vi "FMS Data Array.vi"() -> (0 "FMS Data Array":string[](array[string]), 2 "Scale":string, 3 "Switch":string)   [LabVIEW 2017]
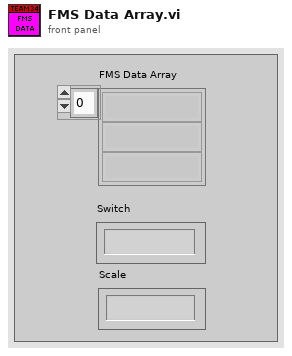
[diagram p1: front panel]
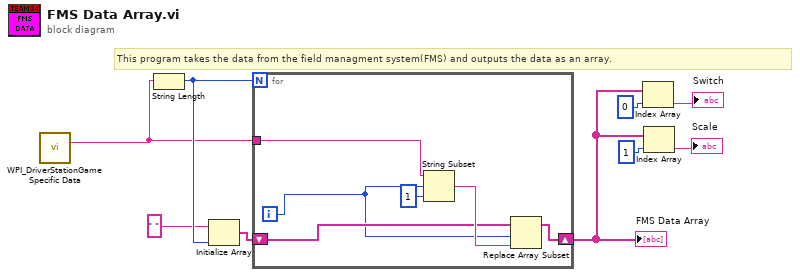
[diagram p0: block diagram]
diagram:
  # "This program takes the data from the field managment system(FMS) and outputs the data as an array."
  n1 = call <vilib>:"WPI_DriverStationGame Specific Data.vi"() -> ("Game Specific Data"=w6:string)  [unwired: 11 in]
  n2 = String Length(string=w6) -> (length=w9:i32)
  n3 = Initialize Array(" ", w9) -> (w7:string[])
  n4 = for {
    N: w9 -> [_]
    shift-right: [w12] -> w3
    shift-left: w7 -> [w13]
    tunnel: w6 -> [w10]
    i -> [w11]
    n5 = String Subset(string=w10, offset (0)=w11, length (rest)=1 ("length (rest)")) -> (substring=w14:string)
    n6 = Replace Array Subset(array=w13, new element=w14, index=w11) -> (w12:string[])
  }
  "FMS Data Array" <- w3
  n7 = Index Array(array=w3, index=0) -> (element=→"Switch":string)
  n8 = Index Array(array=w3, index=1) -> (element=→"Scale":string)
